vi "Leprechaun Program FINAL.vi"   [LabVIEW 2016]
uses:
  <vilib>/NXT/Block Support/NXT_InputPort.ctl
  <vilib>/NXT/Block Support/NXT_OutputPort.ctl
  <vilib>/NXT/Subs/MotorOutput.ctl
  <vilib>/NXT/Dual Mode Library/Sensors/Sonar_cm.vi
  <vilib>/NXT/Dual Mode Library/Sensors/Sound_dB.vi
  <vilib>/NXT/Dual Mode Library/Sensors/Touch_Pressed.vi
  <vilib>/NXT/NXTIO Xnodes/NXTIONodeSubVIs/NXTStopMotors.vi
  <vilib>/NXT/Dual Mode Library/Display/clearDisplay.vi
  <vilib>/NXT/Dual Mode Library/Display/drawText.vi
  <vilib>/NXT/NXTIO Xnodes/NXTIONodeSubVIs/NXTMoveMotors.vi
  <vilib>/NXT/Dual Mode Library/Motors/ResetMotor.vi
  <vilib>/NXT/Dual Mode Library/Waits/Wait_Rotation.vi
  <vilib>/NXT/Dual Mode Library/Waits/Wait_Num.vi
  <vilib>/NXT/Dual Mode Library/Sound/Tone.vi
  <vilib>/NXT/Subs/LVHSConnector.ctl
  <vilib>/NXT/NXTIO Xnodes/AddressXNode/NXTIOAddress.xnode
  <vilib>/NXT/NXTIO Xnodes/NXTIOXNode/NXTIO.xnode
  <vilib>/NXT/LegoClasses/BrickReference/BrickReference.lvclass
types:
  T1 = typedef "NXT_OutputPort.ctl" = u8
  T2 = cluster{"Output Port":T1, "Output Port 2":T1, "Output Port 3":T1}
  T3 = typedef "NXT_InputPort.ctl" = u32
  T4 = typedef "LVHSConnector.ctl" = refnum<class "BrickReference.lvclass">
  T5 = typedef "MotorOutput.ctl" = u8
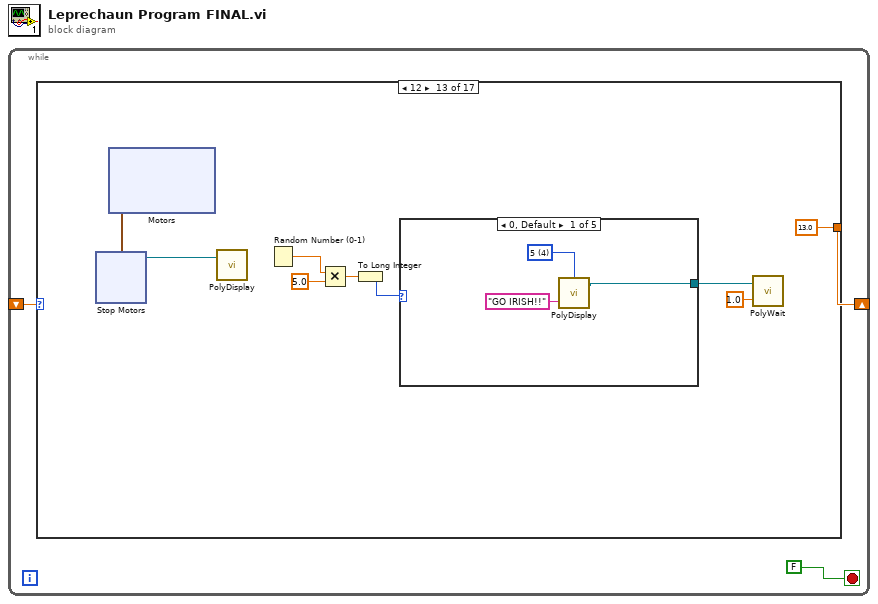
[diagram p0: block diagram]
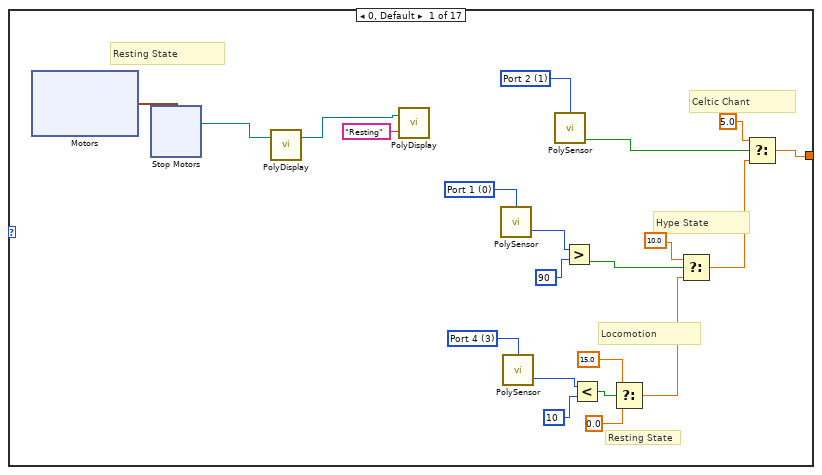
[diagram p2: hidden frame]
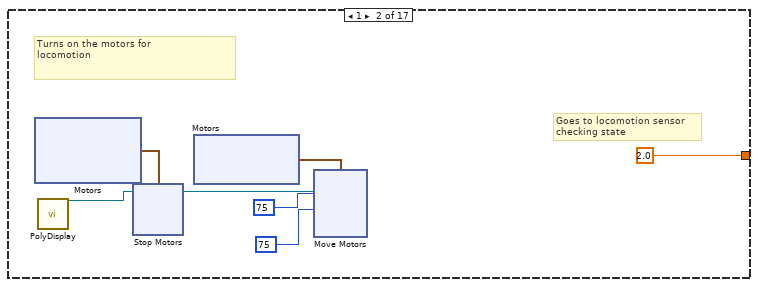
[diagram p3: hidden frame]
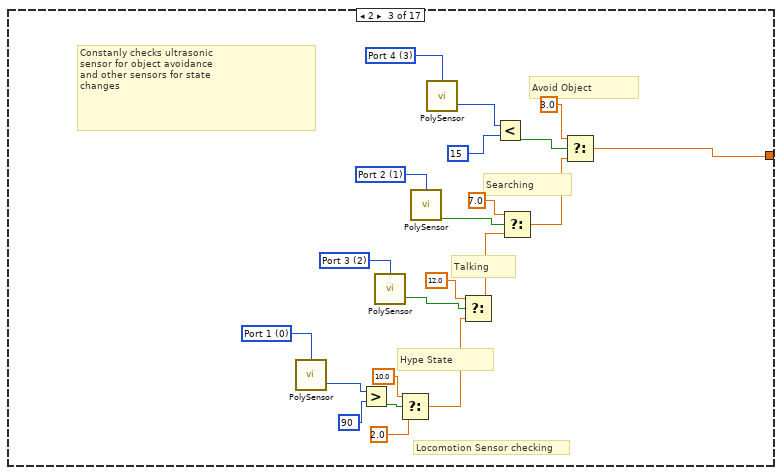
[diagram p4: hidden frame]
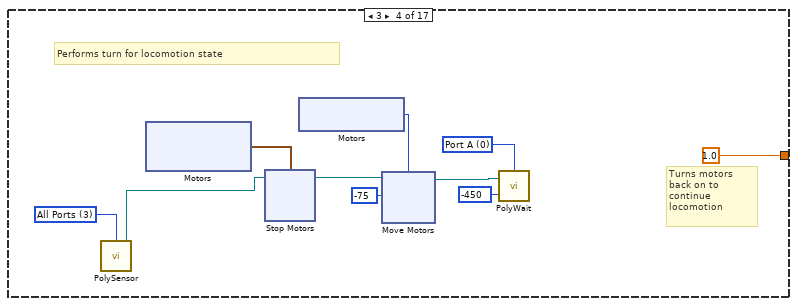
[diagram p5: hidden frame]
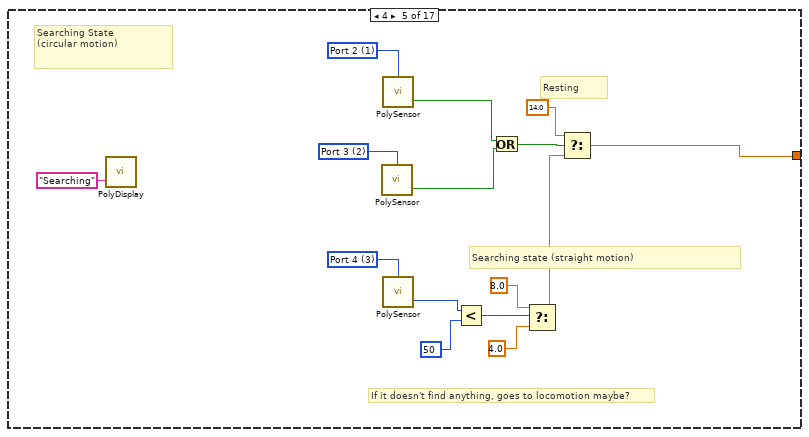
[diagram p6: hidden frame]
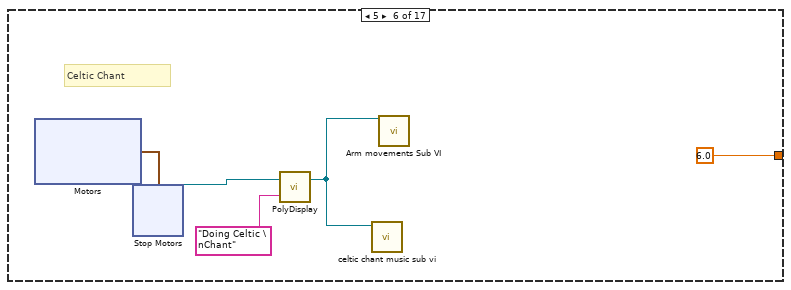
[diagram p7: hidden frame]
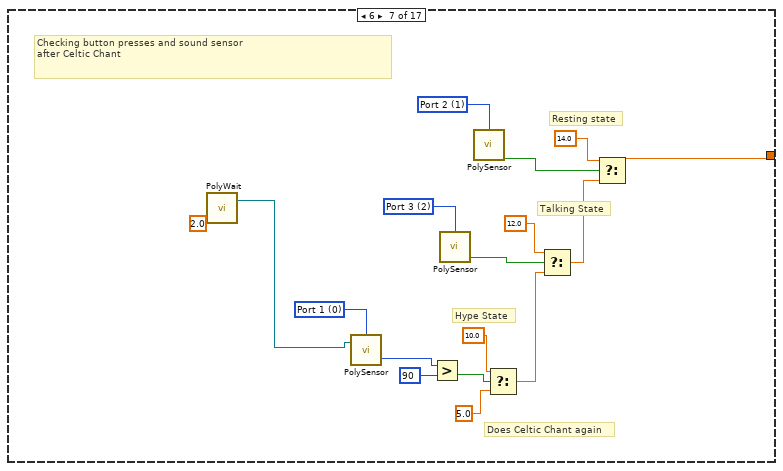
[diagram p8: hidden frame]
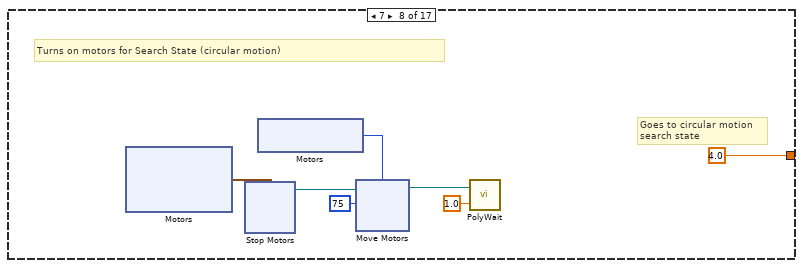
[diagram p9: hidden frame]
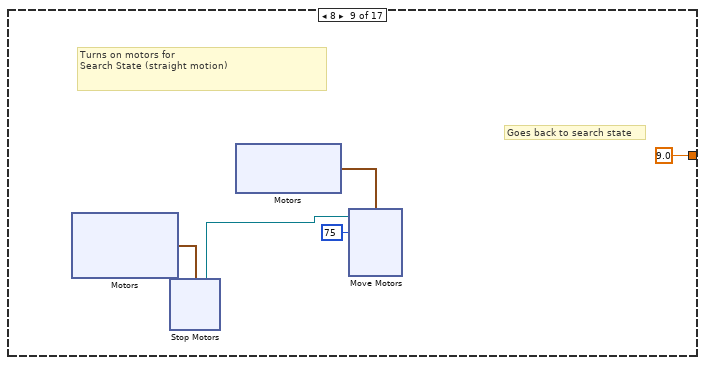
[diagram p10: hidden frame]
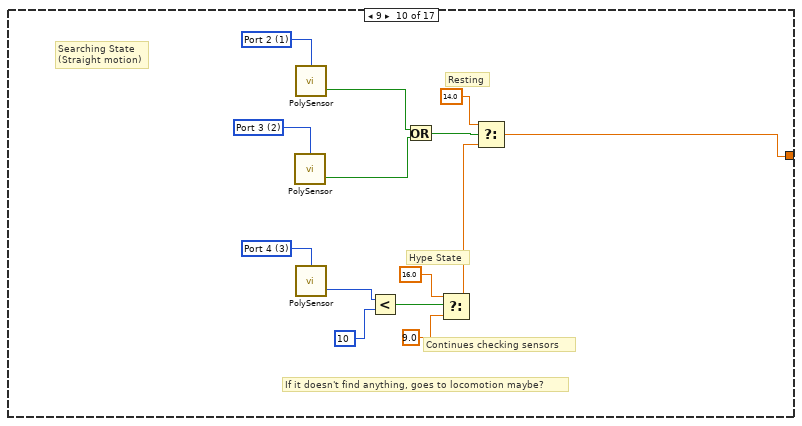
[diagram p11: hidden frame]
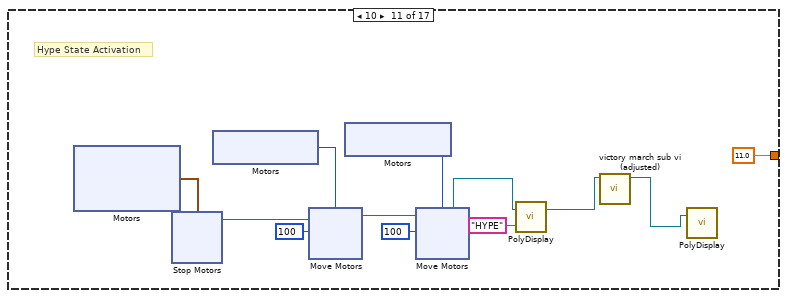
[diagram p12: hidden frame]
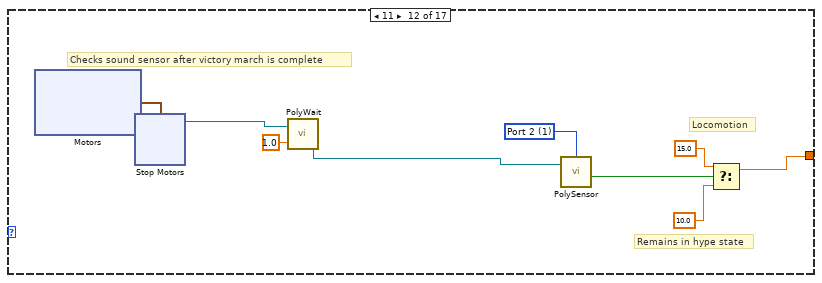
[diagram p13: hidden frame]
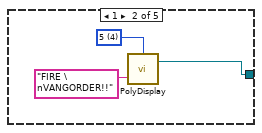
[diagram p14: hidden frame]
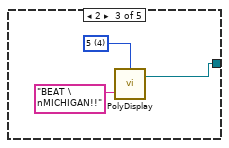
[diagram p15: hidden frame]
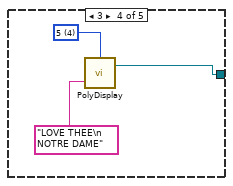
[diagram p16: hidden frame]
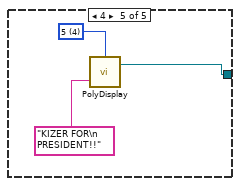
[diagram p17: hidden frame]
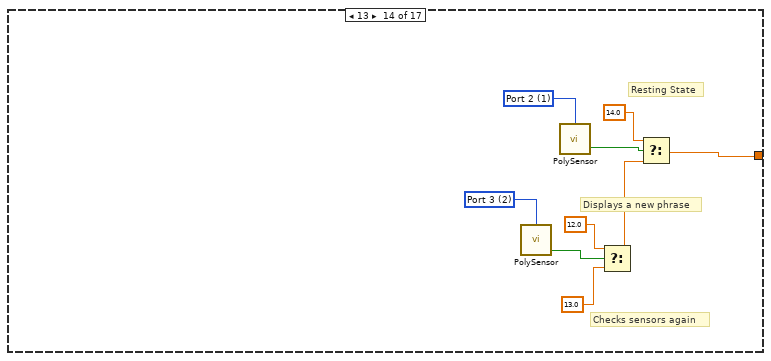
[diagram p18: hidden frame]
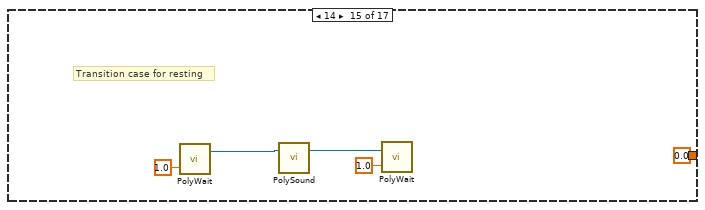
[diagram p19: hidden frame]
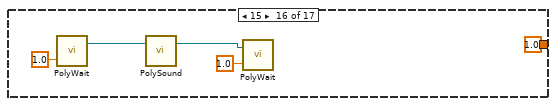
[diagram p20: hidden frame]
diagram:
  n1 = while {
    shift-right: [w3] -> _
    shift-left: _ -> [w2]
    stop <- FALSE stop-if-true
    n2 = case shown="12" w2 {
      tunnel: [w8 2.0 ("f") w53 1.0 ("f") w99 6.0 ("f") w126 4.0 ("f") 9.0 ("f") w182 11.0 ("f") w238 13.0 ("f") w275 0.0 ("f") 1.0 ("f") 10.0 ("f")] -> w3
      frame 0, Default {
        w22 = T3 1 items=["Port 1", "Port 2", "Port 3", "Port 4"] ("Port (Port 1)")
        w23 = T3 0 items=["Port 1", "Port 2", "Port 3", "Port 4"] ("Port (Port 2)")
        w24 = T3 3 items=["Port 1", "Port 2", "Port 3", "Port 4"] ("Port (Port 4)")
        # "Resting State"
        # "Locomotion"
        # "Hype State"
        # "Celtic Chant"
        # "Resting State"
        n3 = xnode "Motors"() -> ("Motor"=w7:cluster{"Port":T1, "Port":T1, "Port":T1})
        n4 = xnode "Stop Motors"("Motors"=w7) -> ("NXT/EV3"=w5:T4)  [unwired: 1 in]
        n5 = call-poly <vilib>:"PolyDisplay.vi"("NXT/EV3"=w5) -> ("NXT/EV3"=w4:T4)  [unwired: 3 in]
        n6 = call-poly <vilib>:"PolyDisplay.vi"("Text"="Resting", "NXT/EV3"=w4) -> ()  [unwired: 2 in, 1 out]
        n7 = call-poly <vilib>:"PolySensor.vi"("Port (Port 2)"=w23) -> ("Sound (dB)"=w19:i16)  [unwired: 2 in, 1 out]
        n8 = call-poly <vilib>:"PolySensor.vi"("Port (Port 4)"=w24) -> ("Distance (cm)"=w14:i16)  [unwired: 2 in, 1 out]
        n9 = call-poly <vilib>:"PolySensor.vi"("Port (Port 1)"=w22) -> ("Yes / No"=w21:bool)  [unwired: 2 in, 1 out]
        n10 = Greater?(x=w19, y=i16 90) -> (0:w17:bool)
        n11 = Less?(x=w14, y=i16 10) -> (x < y?=w12:bool)
        n12 = Select(t=15.0, s=w12, f=0.0) -> (s? t:f=w9:dbl)
        n13 = Select(t=10.0, s=w17, f=w9) -> (s? t:f=w15:dbl)
        n14 = Select(t=5.0, s=w21, f=w15) -> (s? t:f=w8:dbl)
      }
      frame 1 {
        # "Goes to locomotion sensor \nchecking state"
        # "Turns on the motors for \nlocomotion"
        n15 = xnode "Motors"() -> ("Motor"=w33:cluster{"Port":T1, "Port":T1, "Port":T1})
        n16 = call-poly <vilib>:"PolyDisplay.vi"() -> ("NXT/EV3"=w31:T4)  [unwired: 4 in]
        n17 = xnode "Stop Motors"("Motors"=w33, "NXT/EV3"=w31) -> ("NXT/EV3"=w32:T4)
        n18 = xnode "Motors"() -> ("Motor"=w37:cluster{"Port":T1, "Port":T1})
        n19 = xnode "Move Motors"("Power/Speed 2"=i8 75, "Power/Speed 1"=i8 75, "Motors"=w37, "NXT/EV3"=w32) -> ()  [unwired: 1 out]
      }
      frame 2 {
        w60 = T3 0 items=["Port 1", "Port 2", "Port 3", "Port 4"] ("Port (Port 1)")
        w64 = T3 2 items=["Port 1", "Port 2", "Port 3", "Port 4"] ("Port (Port 1)")
        w68 = T3 1 items=["Port 1", "Port 2", "Port 3", "Port 4"] ("Port (Port 1)")
        w73 = T3 3 items=["Port 1", "Port 2", "Port 3", "Port 4"] ("Port (Port 4)")
        # "Locomotion Sensor checking"
        # "Hype State"
        # "Talking"
        # "Searching"
        # "Avoid Object"
        # "Constanly checks ultrasonic \nsensor for object avoidance\nand other sensors for state\nchanges"
        n20 = call-poly <vilib>:"PolySensor.vi"("Port (Port 2)"=w60) -> ("Sound (dB)"=w59:i16)  [unwired: 2 in, 1 out]
        n21 = Greater?(x=w59, y=i16 90) -> (0:w57:bool)
        n22 = call-poly <vilib>:"PolySensor.vi"("Port (Port 1)"=w64) -> ("Yes / No"=w63:bool)  [unwired: 2 in, 1 out]
        n23 = Select(t=10.0, s=w57, f=2.0) -> (s? t:f=w54:dbl)
        n24 = call-poly <vilib>:"PolySensor.vi"("Port (Port 1)"=w68) -> ("Yes / No"=w67:bool)  [unwired: 2 in, 1 out]
        n25 = call-poly <vilib>:"PolySensor.vi"("Port (Port 4)"=w73) -> ("Distance (cm)"=w72:i16)  [unwired: 2 in, 1 out]
        n26 = Select(t=12.0, s=w63, f=w54) -> (s? t:f=w61:dbl)
        n27 = Less?(x=w72, y=i16 15) -> (x < y?=w70:bool)
        n28 = Select(t=7.0, s=w67, f=w61) -> (s? t:f=w65:dbl)
        n29 = Select(t=3.0, s=w70, f=w65) -> (s? t:f=w53:dbl)
      }
      frame 3 {
        w74 = T5 3 items=["Port A"=0, "Port B"=1, "Port C"=2, "Ports A & B"=4, "Ports A & C"=5, "Ports B & C"=6, "All Ports"=3] ("Port (All Ports)")
        w76 = T1 0 items=["Port A", "Port B", "Port C", "Port D"] ("Port (Port A)")
        # "Turns motors\nback on to continue locomotion"
        # "Performs turn for locomotion state"
        n30 = call-poly <vilib>:"PolySensor.vi"("Port (All Ports)"=w74) -> ("NXT/EV3"=w80:T4)  [unwired: 3 in]
        n31 = xnode "Motors"() -> ("Motor"=w83:cluster{"Port":T1, "Port":T1})
        n32 = xnode "Stop Motors"("Motors"=w83, "NXT/EV3"=w80) -> ("NXT/EV3"=w82:T4)
        n33 = xnode "Motors"() -> ("Motor"=w81:T1)
        n34 = xnode "Move Motors"("Power/Speed 1"=i8 -75, "Motors"=w81, "NXT/EV3"=w82) -> ("NXT/EV3"=w78:T4)
        n35 = call-poly <vilib>:"PolyWait.vi"("Position Change (180)"=-450, "NXT/EV3"=w78, "Port (Port A)"=w76) -> ()  [unwired: 1 in, 1 out]
      }
      frame 4 {
        w106 = T3 3 items=["Port 1", "Port 2", "Port 3", "Port 4"] ("Port (Port 4)")
        w111 = T3 2 items=["Port 1", "Port 2", "Port 3", "Port 4"] ("Port (Port 1)")
        w112 = T3 1 items=["Port 1", "Port 2", "Port 3", "Port 4"] ("Port (Port 1)")
        # "If it doesn't find anything, goes to locomotion maybe?"
        # "Searching state (straight motion)"
        # "Resting"
        # "Searching State\n(circular motion)"
        n36 = call-poly <vilib>:"PolyDisplay.vi"("Text"="Searching") -> ()  [unwired: 3 in, 1 out]
        n37 = call-poly <vilib>:"PolySensor.vi"("Port (Port 1)"=w111) -> ("Yes / No"=w109:bool)  [unwired: 2 in, 1 out]
        n38 = call-poly <vilib>:"PolySensor.vi"("Port (Port 1)"=w112) -> ("Yes / No"=w110:bool)  [unwired: 2 in, 1 out]
        n39 = call-poly <vilib>:"PolySensor.vi"("Port (Port 4)"=w106) -> ("Distance (cm)"=w105:i16)  [unwired: 2 in, 1 out]
        n40 = Less?(x=w105, y=i16 50) -> (x < y?=w103:bool)
        n41 = Or(x=w110, y=w109) -> (x .or. y?=w108:bool)
        n42 = Select(t=8.0, s=w103, f=4.0) -> (s? t:f=w100:dbl)
        n43 = Select(t=14.0, s=w108, f=w100) -> (s? t:f=w99:dbl)
      }
      frame 5 {
        # "Celtic Chant"
        n44 = xnode "Motors"() -> ("Motor"=w116:cluster{"Port":T1, "Port":T1, "Port":T1})
        n45 = xnode "Stop Motors"("Motors"=w116) -> ("NXT/EV3"=w115:T4)  [unwired: 1 in]
        n46 = call-poly <vilib>:"PolyDisplay.vi"("Text"="Doing Celtic \nChant", "NXT/EV3"=w115) -> ("NXT/EV3"=w113:T4)  [unwired: 2 in]
        n47 = call "celtic chant music sub vi.vi"("BrickReference in"=w113) -> ()  [unwired: 10 in, 1 out]
        n48 = call "Arm movements Sub VI.vi"("BrickReference in"=w113) -> ()  [unwired: 10 in, 1 out]
      }
      frame 6 {
        w133 = T3 0 items=["Port 1", "Port 2", "Port 3", "Port 4"] ("Port (Port 1)")
        w137 = T3 2 items=["Port 1", "Port 2", "Port 3", "Port 4"] ("Port (Port 1)")
        w139 = T3 1 items=["Port 1", "Port 2", "Port 3", "Port 4"] ("Port (Port 1)")
        # "Does Celtic Chant again"
        # "Hype State"
        # "Talking State"
        # "Resting state"
        # "Checking button presses and sound sensor\nafter Celtic Chant"
        n49 = call-poly <vilib>:"PolyWait.vi"("Time (1 sec)"=sgl 2.0) -> ("NXT/EV3"=w124:T4)  [unwired: 3 in]
        n50 = call-poly <vilib>:"PolySensor.vi"("NXT/EV3"=w124, "Port (Port 2)"=w133) -> ("Sound (dB)"=w132:i16)  [unwired: 1 in, 1 out]
        n51 = Greater?(x=w132, y=i16 90) -> (0:w130:bool)
        n52 = call-poly <vilib>:"PolySensor.vi"("Port (Port 1)"=w137) -> ("Yes / No"=w136:bool)  [unwired: 2 in, 1 out]
        n53 = call-poly <vilib>:"PolySensor.vi"("Port (Port 1)"=w139) -> ("Yes / No"=w140:bool)  [unwired: 2 in, 1 out]
        n54 = Select(t=10.0, s=w130, f=5.0) -> (s? t:f=w127:dbl)
        n55 = Select(t=12.0, s=w136, f=w127) -> (s? t:f=w135:dbl)
        n56 = Select(t=14.0, s=w140, f=w135) -> (s? t:f=w126:dbl)
      }
      frame 7 {
        # "Goes to circular motion \nsearch state"
        # "Turns on motors for Search State (circular motion)"
        n57 = xnode "Motors"() -> ("Motor"=w146:cluster{"Port":T1, "Port":T1, "Port":T1})
        n58 = xnode "Stop Motors"("Motors"=w146) -> ("NXT/EV3"=w145:T4)  [unwired: 1 in]
        n59 = xnode "Motors"() -> ("Motor"=w143:T1)
        n60 = xnode "Move Motors"("Power/Speed 1"=i8 75, "Motors"=w143, "NXT/EV3"=w145) -> ("NXT/EV3"=w142:T4)
        n61 = call-poly <vilib>:"PolyWait.vi"("Time (1 sec)"=sgl 1.0, "NXT/EV3"=w142) -> ()  [unwired: 2 in, 1 out]
      }
      frame 8 {
        # "Goes back to search state"
        # "Turns on motors for\nSearch State (straight motion)"
        n62 = xnode "Motors"() -> ("Motor"=w163:cluster{"Port":T1, "Port":T1, "Port":T1})
        n63 = xnode "Stop Motors"("Motors"=w163) -> ("NXT/EV3"=w162:T4)  [unwired: 1 in]
        n64 = xnode "Motors"() -> ("Motor"=w165:cluster{"Port":T1, "Port":T1})
        n65 = xnode "Move Motors"("Power/Speed 1"=i8 75, "Motors"=w165, "NXT/EV3"=w162) -> ()  [unwired: 1 in, 1 out]
      }
      frame 9 {
        w189 = T3 3 items=["Port 1", "Port 2", "Port 3", "Port 4"] ("Port (Port 4)")
        w194 = T3 2 items=["Port 1", "Port 2", "Port 3", "Port 4"] ("Port (Port 1)")
        w195 = T3 1 items=["Port 1", "Port 2", "Port 3", "Port 4"] ("Port (Port 1)")
        # "Resting"
        # "Searching State\n(Straight motion)"
        # "Continues checking sensors"
        # "Hype State"
        # "If it doesn't find anything, goes to locomotion maybe?"
        n66 = call-poly <vilib>:"PolySensor.vi"("Port (Port 1)"=w194) -> ("Yes / No"=w192:bool)  [unwired: 2 in, 1 out]
        n67 = call-poly <vilib>:"PolySensor.vi"("Port (Port 1)"=w195) -> ("Yes / No"=w193:bool)  [unwired: 2 in, 1 out]
        n68 = call-poly <vilib>:"PolySensor.vi"("Port (Port 4)"=w189) -> ("Distance (cm)"=w188:i16)  [unwired: 2 in, 1 out]
        n69 = Less?(x=w188, y=i16 10) -> (x < y?=w186:bool)
        n70 = Or(x=w193, y=w192) -> (x .or. y?=w191:bool)
        n71 = Select(t=16.0, s=w186, f=9.0) -> (s? t:f=w183:dbl)
        n72 = Select(t=14.0, s=w191, f=w183) -> (s? t:f=w182:dbl)
      }
      frame 10 {
        # "Hype State Activation"
        n73 = xnode "Motors"() -> ("Motor"=w207:cluster{"Port":T1, "Port":T1, "Port":T1})
        n74 = xnode "Stop Motors"("Motors"=w207) -> ("NXT/EV3"=w206:T4)  [unwired: 1 in]
        n75 = xnode "Motors"() -> ("Motor"=w205:T1)
        n76 = xnode "Move Motors"("Power/Speed 1"=i8 100, "Motors"=w205, "NXT/EV3"=w206) -> ("NXT/EV3"=w203:T4)
        n77 = xnode "Motors"() -> ("Motor"=w201:T1)
        n78 = xnode "Move Motors"("Power/Speed 1"=i8 100, "Motors"=w201, "NXT/EV3"=w203) -> ("NXT/EV3"=w199:T4)
        n79 = call-poly <vilib>:"PolyDisplay.vi"("Text"="HYPE", "NXT/EV3"=w199) -> ("NXT/EV3"=w196:T4)  [unwired: 2 in]
        n80 = call "victory march sub vi (adjusted).vi"("BrickReference in"=w196) -> ("BrickReference out"=w197:T4)  [unwired: 10 in]
        n81 = call-poly <vilib>:"PolyDisplay.vi"("NXT/EV3"=w197) -> ()  [unwired: 3 in, 1 out]
      }
      frame 11 {
        w234 = T3 1 items=["Port 1", "Port 2", "Port 3", "Port 4"] ("Port (Port 1)")
        # "Checks sound sensor after victory march is complete"
        # "Remains in hype state"
        # "Locomotion"
        n82 = xnode "Motors"() -> ("Motor"=w230:cluster{"Port":T1, "Port":T1, "Port":T1})
        n83 = xnode "Stop Motors"("Motors"=w230) -> ("NXT/EV3"=w231:T4)  [unwired: 1 in]
        n84 = call-poly <vilib>:"PolyWait.vi"("Time (1 sec)"=sgl 1.0, "NXT/EV3"=w231) -> ("NXT/EV3"=w232:T4)  [unwired: 2 in]
        n85 = call-poly <vilib>:"PolySensor.vi"("NXT/EV3"=w232, "Port (Port 1)"=w234) -> ("Yes / No"=w233:bool)  [unwired: 1 in, 1 out]
        n86 = Select(t=15.0, s=w233, f=10.0) -> (s? t:f=w238:dbl)
      }
      frame 12 {
        n87 = xnode "Motors"() -> ("Motor"=w251:cluster{"Port":T1, "Port":T1, "Port":T1})
        n88 = xnode "Stop Motors"("Motors"=w251) -> ("NXT/EV3"=w249:T4)  [unwired: 1 in]
        n89 = call-poly <vilib>:"PolyDisplay.vi"("NXT/EV3"=w249) -> ()  [unwired: 3 in, 1 out]
        n90 = Random Number (0-1)() -> (number: 0 to 1=w250:dbl)
        n91 = Multiply(x=w250, y=5.0) -> (x*y=w248:dbl)
        n92 = To Long Integer(number=w248) -> (32bit integer=w247:i32)
        n93 = case shown="0, Default" w247 {
          tunnel: [w261 w264 w267 w270 w273] -> w246
          frame 0, Default {
            w260 = i16 4 items=["1", "2", "3", "4", "5", "6", "7", "8", "9", "10", "11", "12"] ("Line")
            n94 = call-poly <vilib>:"PolyDisplay.vi"("Text"="GO IRISH!!", "Line"=w260) -> ("NXT/EV3"=w261:T4)  [unwired: 2 in]
          }
          frame 1 {
            w263 = i16 4 items=["1", "2", "3", "4", "5", "6", "7", "8", "9", "10", "11", "12"] ("Line")
            n95 = call-poly <vilib>:"PolyDisplay.vi"("Text"="FIRE \nVANGORDER!!", "Line"=w263) -> ("NXT/EV3"=w264:T4)  [unwired: 2 in]
          }
          frame 2 {
            w266 = i16 4 items=["1", "2", "3", "4", "5", "6", "7", "8", "9", "10", "11", "12"] ("Line")
            n96 = call-poly <vilib>:"PolyDisplay.vi"("Text"="BEAT \nMICHIGAN!!", "Line"=w266) -> ("NXT/EV3"=w267:T4)  [unwired: 2 in]
          }
          frame 3 {
            w269 = i16 4 items=["1", "2", "3", "4", "5", "6", "7", "8", "9", "10", "11", "12"] ("Line")
            n97 = call-poly <vilib>:"PolyDisplay.vi"("Text"="LOVE THEE\n NOTRE DAME", "Line"=w269) -> ("NXT/EV3"=w270:T4)  [unwired: 2 in]
          }
          frame 4 {
            w272 = i16 4 items=["1", "2", "3", "4", "5", "6", "7", "8", "9", "10", "11", "12"] ("Line")
            n98 = call-poly <vilib>:"PolyDisplay.vi"("Text"="KIZER FOR\n PRESIDENT!!", "Line"=w272) -> ("NXT/EV3"=w273:T4)  [unwired: 2 in]
          }
        }
        n99 = call-poly <vilib>:"PolyWait.vi"("Time (1 sec)"=sgl 1.0, "NXT/EV3"=w246) -> ()  [unwired: 2 in, 1 out]
      }
      frame 13 {
        w280 = T3 2 items=["Port 1", "Port 2", "Port 3", "Port 4"] ("Port (Port 1)")
        w283 = T3 1 items=["Port 1", "Port 2", "Port 3", "Port 4"] ("Port (Port 1)")
        # "Checks sensors again"
        # "Displays a new phrase"
        # "Resting State"
        n100 = call-poly <vilib>:"PolySensor.vi"("Port (Port 1)"=w280) -> ("Yes / No"=w279:bool)  [unwired: 2 in, 1 out]
        n101 = call-poly <vilib>:"PolySensor.vi"("Port (Port 1)"=w283) -> ("Yes / No"=w282:bool)  [unwired: 2 in, 1 out]
        n102 = Select(t=12.0, s=w279, f=13.0) -> (s? t:f=w276:dbl)
        n103 = Select(t=14.0, s=w282, f=w276) -> (s? t:f=w275:dbl)
      }
      frame 14 {
        # "Transition case for resting"
        n104 = call-poly <vilib>:"PolyWait.vi"("Time (1 sec)"=sgl 1.0) -> ("NXT/EV3"=w286:T4)  [unwired: 3 in]
        n105 = call-poly <vilib>:"PolySound.vi"("NXT/EV3"=w286) -> ("NXT/EV3"=w285:T4)  [unwired: 3 in]
        n106 = call-poly <vilib>:"PolyWait.vi"("Time (1 sec)"=sgl 1.0, "NXT/EV3"=w285) -> ()  [unwired: 2 in, 1 out]
      }
      frame 15 {
        n107 = call-poly <vilib>:"PolyWait.vi"("Time (1 sec)"=sgl 1.0) -> ("NXT/EV3"=w292:T4)  [unwired: 3 in]
        n108 = call-poly <vilib>:"PolySound.vi"("NXT/EV3"=w292) -> ("NXT/EV3"=w291:T4)  [unwired: 3 in]
        n109 = call-poly <vilib>:"PolyWait.vi"("Time (1 sec)"=sgl 1.0, "NXT/EV3"=w291) -> ()  [unwired: 2 in, 1 out]
      }
      frame 16 {
        n110 = xnode "Motors"() -> ("Motor"=w301:cluster{"Port":T1, "Port":T1})
        n111 = xnode "Move Motors"("Power/Speed 2"=i8 -75, "Power/Speed 1"=i8 -75, "Motors"=w301) -> ("NXT/EV3"=w298:T4)  [unwired: 1 in]
        n112 = call-poly <vilib>:"PolyWait.vi"("Time (1 sec)"=sgl 1.0, "NXT/EV3"=w298) -> ("NXT/EV3"=w296:T4)  [unwired: 2 in]
        n113 = xnode "Motors"() -> ("Motor"=w295:cluster{"Port":T1, "Port":T1})
        n114 = xnode "Stop Motors"("Motors"=w295, "NXT/EV3"=w296) -> ()  [unwired: 1 out]
      }
    }
  }
